vi "Get State.vi"(8 "error in (no error)":errorcluster, 11 "Pulse Controller in":refnum<class "Channel Scanner.lvclass">) -> (0 "error out":errorcluster, 1 "Result ready":bool, 2 "Armed":bool, 3 "Pulse Controller out":refnum<class "Channel Scanner.lvclass">)   [LabVIEW 2016, in "Channel Scanner.lvclass"]
uses:
  Channel Scanner.lvclass
  Channel Scanner.lvclass/Channel Scanner.ctl
  Instrument Actor/Instrument Actor.lvclass
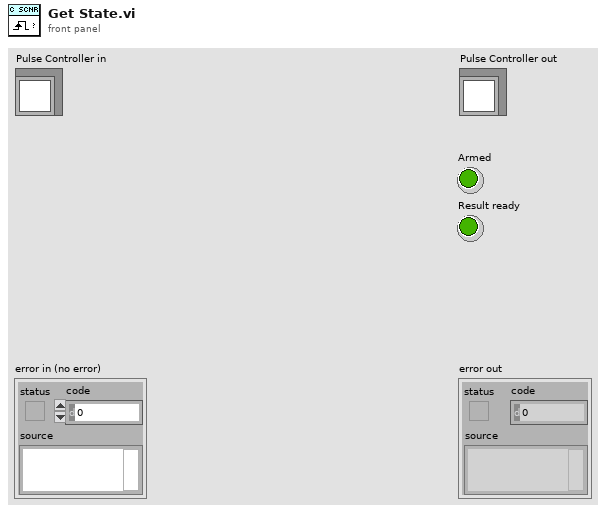
[diagram p1: front panel]
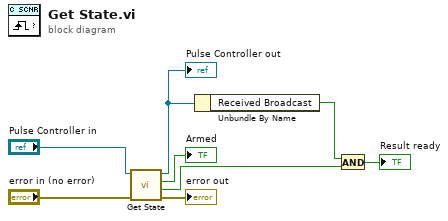
[diagram p0: block diagram]
diagram:
  n1 = call-parent "Get State.vi"("error in (no error)"="error in (no error)", "Pulse Controller in"="Pulse Controller in") -> ("error out"=→"error out":errorcluster, "Result ready"=w3:bool, "Armed"=→"Armed":bool, "Pulse Controller out"=w4:refnum<class "Channel Scanner.lvclass">)  [unwired: 6 in]
  "Pulse Controller out" <- w4
  n2 = Unbundle By Name(w4) -> ("Received Broadcast"=w2:bool)
  n3 = And(x=w2, y=w3) -> (x .and. y?=→"Result ready":bool)
